vi "Catch.vi"(11 "Joystick Data":T1) -> (0 "Finished":bool=TRUE, 1 "Arm finger state":T2, 2 "Roller Speed":dbl)   [LabVIEW 2013]
uses:
  <vilib>/Rock Robotics/WPI/Solenoid/WPI_SolenoidValue.ctl
  Joystick Data.ctl
  Catch States.ctl
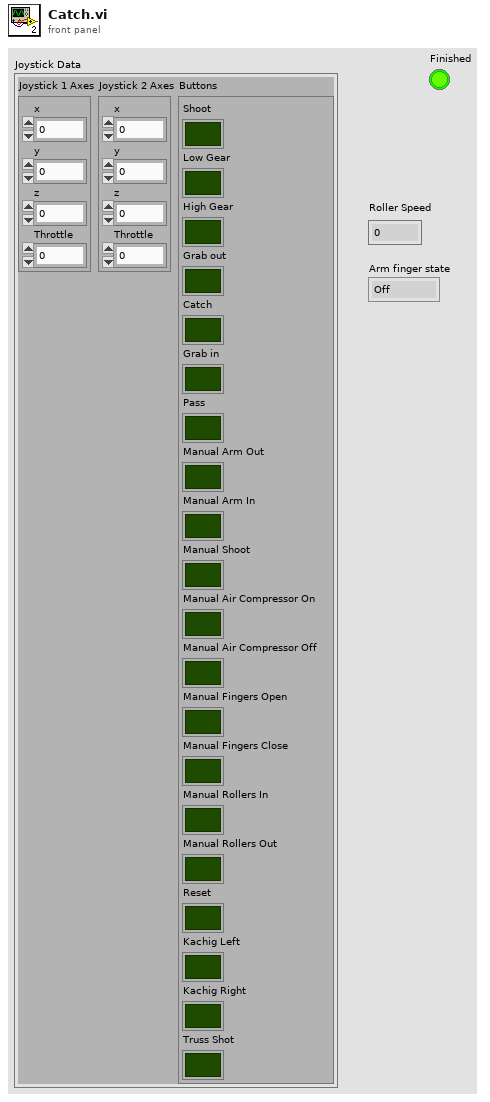
[diagram p1: front panel]
types:
  T1 = typedef "Joystick Data.ctl" = cluster{"Joystick 1 Axes":cluster{"x":dbl, "y":dbl, "z":dbl, "Throttle":dbl}, "Joystick 2 Axes":cluster{"x":dbl, "y":dbl, "z":dbl, "Throttle":dbl}, "Buttons":cluster{"Shoot":bool, "Low Gear":bool, "High Gear":bool, "Grab out":bool, "Catch":bool, "Grab in":bool, "Pass":bool, "Manual Arm Out":bool, "Manual Arm In":bool, "Manual Shoot":bool, "Manual Air Compressor On":bool, "Manual Air Compressor Off":bool, "Manual Fingers Open":bool, "Manual Fingers Close":bool, "Manual Rollers In":bool, "Manual Rollers Out":bool, "Reset":bool, "Kachig Left":bool, "Kachig Right":bool, "Truss Shot":bool}}
  T2 = typedef "WPI_SolenoidValue.ctl" = enum16{"Off", "On", "Forward", "Reverse"}
  T3 = typedef "Catch States.ctl" = enum16{"Catch", "Grab", "Finished"}
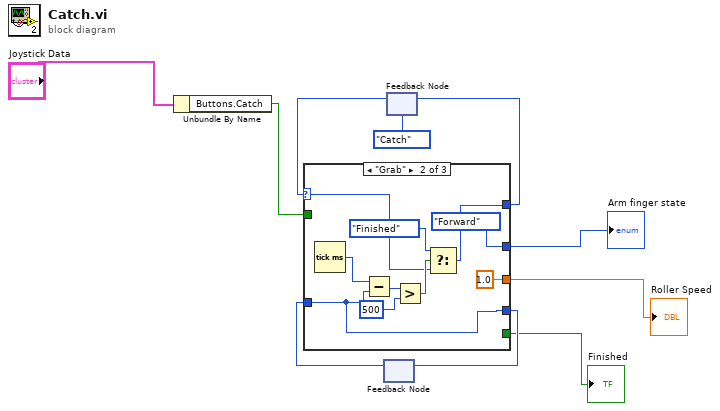
[diagram p0: block diagram]
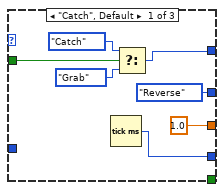
[diagram p2: hidden frame]
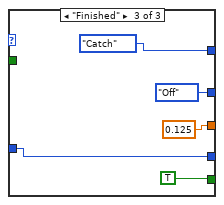
[diagram p3: hidden frame]
diagram:
  n1 = Unbundle By Name("Joystick Data") -> ("Buttons.Catch"=w8:bool)
  n2 = feedback #1() -> (w6:u32)  [unwired: 1 in]
  n3 = feedback #2(Catch_States."Catch") -> (w5:T3)
  n4 = case shown="\"Grab\"" w5 {
    selector: w5 -> [_ w23 _]
    tunnel: [w14 w21 Catch_States."Catch"] -> w4
    tunnel: w8 -> [w17 _ _]
    tunnel: [w16 w18 w29] -> w7
    tunnel: w6 -> [_ w18 w29]
    tunnel: [WPI_SolenoidValue."Reverse" ("Arm State") WPI_SolenoidValue."Forward" ("Arm State") WPI_SolenoidValue."Off" ("Arm State")] -> w1
    tunnel: [1.0 ("Roller Speed") 1.0 ("Roller Speed") 0.125] -> w3
    tunnel: [_ _ TRUE] -> w2
    frame "Catch", Default {
      n5 = Tick Count (ms)() -> (millisecond timer value=w16:u32)
      n6 = Select(t=Catch_States."Catch" ("f"), s=w17, f=Catch_States."Grab") -> (s? t:f=w14:T3)
    }
    frame "Grab" {
      n7 = Tick Count (ms)() -> (millisecond timer value=w27:u32)
      n8 = Subtract(x=w27, y=w18) -> (x-y=w26:u32)
      n9 = Greater?(x=w26, y=500) -> (0:w24:bool)
      n10 = Select(t=Catch_States."Finished", s=w24, f=w23) -> (s? t:f=w21:T3)
    }
    frame "Finished" {
    }
  }
  "Arm finger state" <- w1
  "Roller Speed" <- w3
  "Finished" <- w2
  n11 = feedback-in #1(w7) -> ()
  n12 = feedback-in #2(w4) -> ()
